vi "Send TDMS Cleanup EMG only.vi"(5 "Accel TDMS File":refnum<k34>, 7 "Priority":T1=enum."Normal" caption="Message Priority (Normal)", 8 "error in (no error)":errorcluster, 9 "Force TDMS File":refnum<k34>, 10 "TDMS File":path, 11 "Message Enqueuer in":refnum<class "Message Enqueuer.lvclass">) -> (0 "error out":errorcluster, 3 "Message Enqueuer out":refnum<class "Message Enqueuer.lvclass">)   [LabVIEW 2020, in "Logging.lvlib" / "TDMS Cleanup EMG only Msg.lvclass"]
doc: "Sends the <b>Logging.lvlib:TDMS Cleanup EMG only Msg.lvclass</b> message.\n\nThis message will call <b>TDMS Cleanup EMG only.vi</b> on the <b>Logging.lvlib:Logging.lvclass</b> actor.\n\n<b>TDMS Cleanup EMG only.vi Description</b>"
uses:
  TDMS Cleanup EMG only Msg.lvclass
  <vilib>/ActorFramework/Message Enqueuer/Message Enqueuer.lvclass
  <vilib>/ActorFramework/Message Enqueuer/Message Priority.ctl
  C:/Program Files/National Instruments/LabVIEW 2020/vi.lib/ActorFramework/Message/Message.lvclass
  TDMS Cleanup EMG only Msg.lvclass/TDMS Cleanup EMG only Msg.ctl
  <vilib>/ActorFramework/Message Enqueuer/Message Enqueuer.lvclass/Message Enqueuer.ctl
  <vilib>/ActorFramework/Message Priority Queue/Priority Enqueue.vi
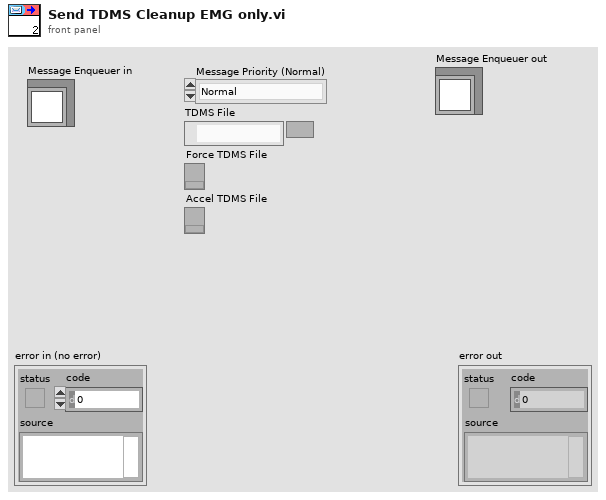
[diagram p1: front panel]
types:
  T1 = typedef "Actor Framework.lvlib/Message Enqueuer.lvclass/Message Priority.ctl" = enum16{"Low", "Normal", "High"}
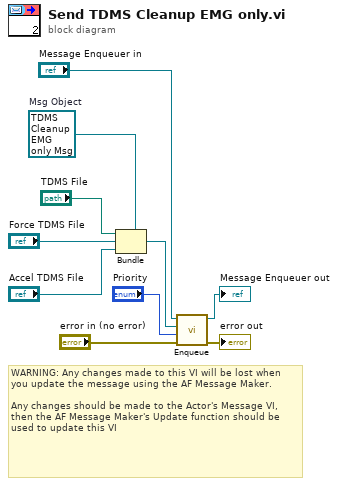
[diagram p0: block diagram]
diagram:
  w7 = refnum<class "TDMS Cleanup EMG only Msg.lvclass"> refnum  # Msg Object
  # "WARNING: Any changes made to this VI will be lost when you update the message using the AF Message Maker.\n\nAny changes should be made to the Actor's Message VI, then the AF Message Maker's Update function should be used to update this VI"
  n1 = Bundle(cluster=w7, "TDMS File", "Force TDMS File", "Accel TDMS File") -> (w2:refnum<class "TDMS Cleanup EMG only Msg.lvclass">)
  n2 = call <vilib>:"Enqueue.vi"("error in (no error)"="error in (no error)", "Message Priority (Normal)"="Priority", "Message"=w2, "Message Enqueuer in"="Message Enqueuer in") -> ("error out"=→"error out":errorcluster, "Message Enqueuer out"=→"Message Enqueuer out":refnum<class "Message Enqueuer.lvclass">)  [unwired: 6 in]
